vi "双路单通通断器（U64）.vi"(7 "默认值":u64, 9 "X直通？":bool=TRUE, 10 "Y_In":u64, 11 "X_In":u64) -> (2 "Y_Out":u64, 3 "X_Out":u64)   [LabVIEW 2013]
doc: "功能：\n\n返回一个枚举，表明输入数的范围，用于三段比较。\n\n\nCSXCS_366创建。"
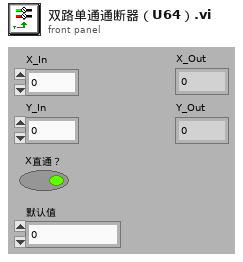
[diagram p1: front panel]
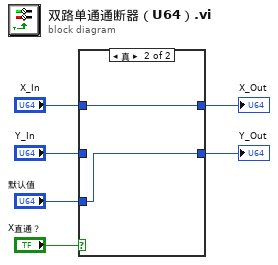
[diagram p0: block diagram]
diagram:
  n1 = case shown="真" "X直通？" {
    tunnel: "X_In" -> [_ w10]
    tunnel: [w8 w10] -> w2
    tunnel: "Y_In" -> [w7 _]
    tunnel: [w7 w9] -> w1
    tunnel: "默认值" -> [w8 w9]
    frame False {
    }
    frame True {
    }
  }
  "X_Out" <- w2
  "Y_Out" <- w1
